vi "measure RTD (host).vi"() -> ()   [LabVIEW 2012]
uses:
  <vilib>/FPGAPlugInAG/PCIe-7852R/niLvFpga_Open_PCIe-7852R.vi
  <vilib>/rvi/interface/common/dynamic/niFpgaDynamicAddResources.vi
  <vilib>/Utility/error.llb/Error Cluster From Error Code.vi
  <vilib>/rvi/errors/niLvFpgaAdjustHostInterfaceError.vi
  <vilib>/rvi/interface/nirviOpenFPGA/nirviOpenFPGA.xnode
  FPGA Bitfiles/UHR-FleezersInst_FPGATarget_rtdmeasure(fpga)_zG2qwe5Jbpg.lvbitx
  rtd measure (fpga).vi
  <vilib>/rvi/interface/nirviReadWriteControl/nirviReadWriteControl.xnode
  NiFpgaLv.dll
  <vilib>/rvi/interface/Simulation/niFpgaSimulationCallBeginRW.vi
panel:
  out "Temp Var":dbl[][](graph) caption="Temperature Variation (F) (initial temp subtracted)"
  out "Absolute Temperature (F)":dbl[][](graph)
  out "Temp (F)":dbl[](array[numeric])
  out "Temp (C)":dbl[](array[numeric])
  out "Resistance":fxp<+/-,24,10>[](array[numeric])
  out "Path Out":path
  out "Index In":dbl=1.0
  in  "Save the data":bool
  in  "stop":bool
  in  "milliseconds to wait":u32=100
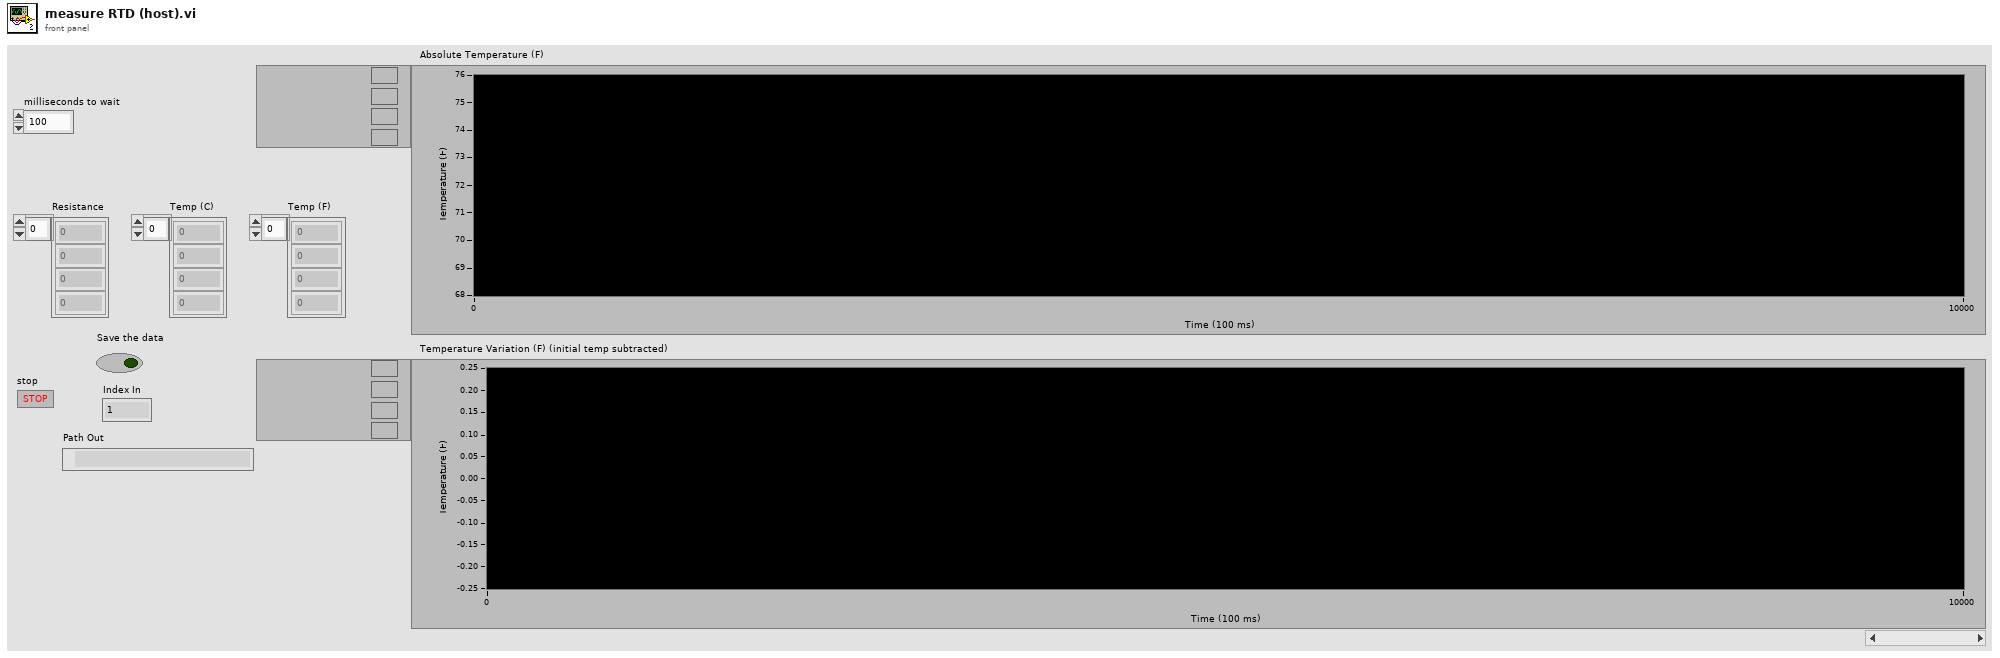
[diagram p1: front panel]
types:
  T1 = enum16{"big-endian, network order", "native, host order", "little-endian"}
  T2 = enum16{"open", "replace", "create", "open or create", "replace or create", "replace or create with confirmation"}
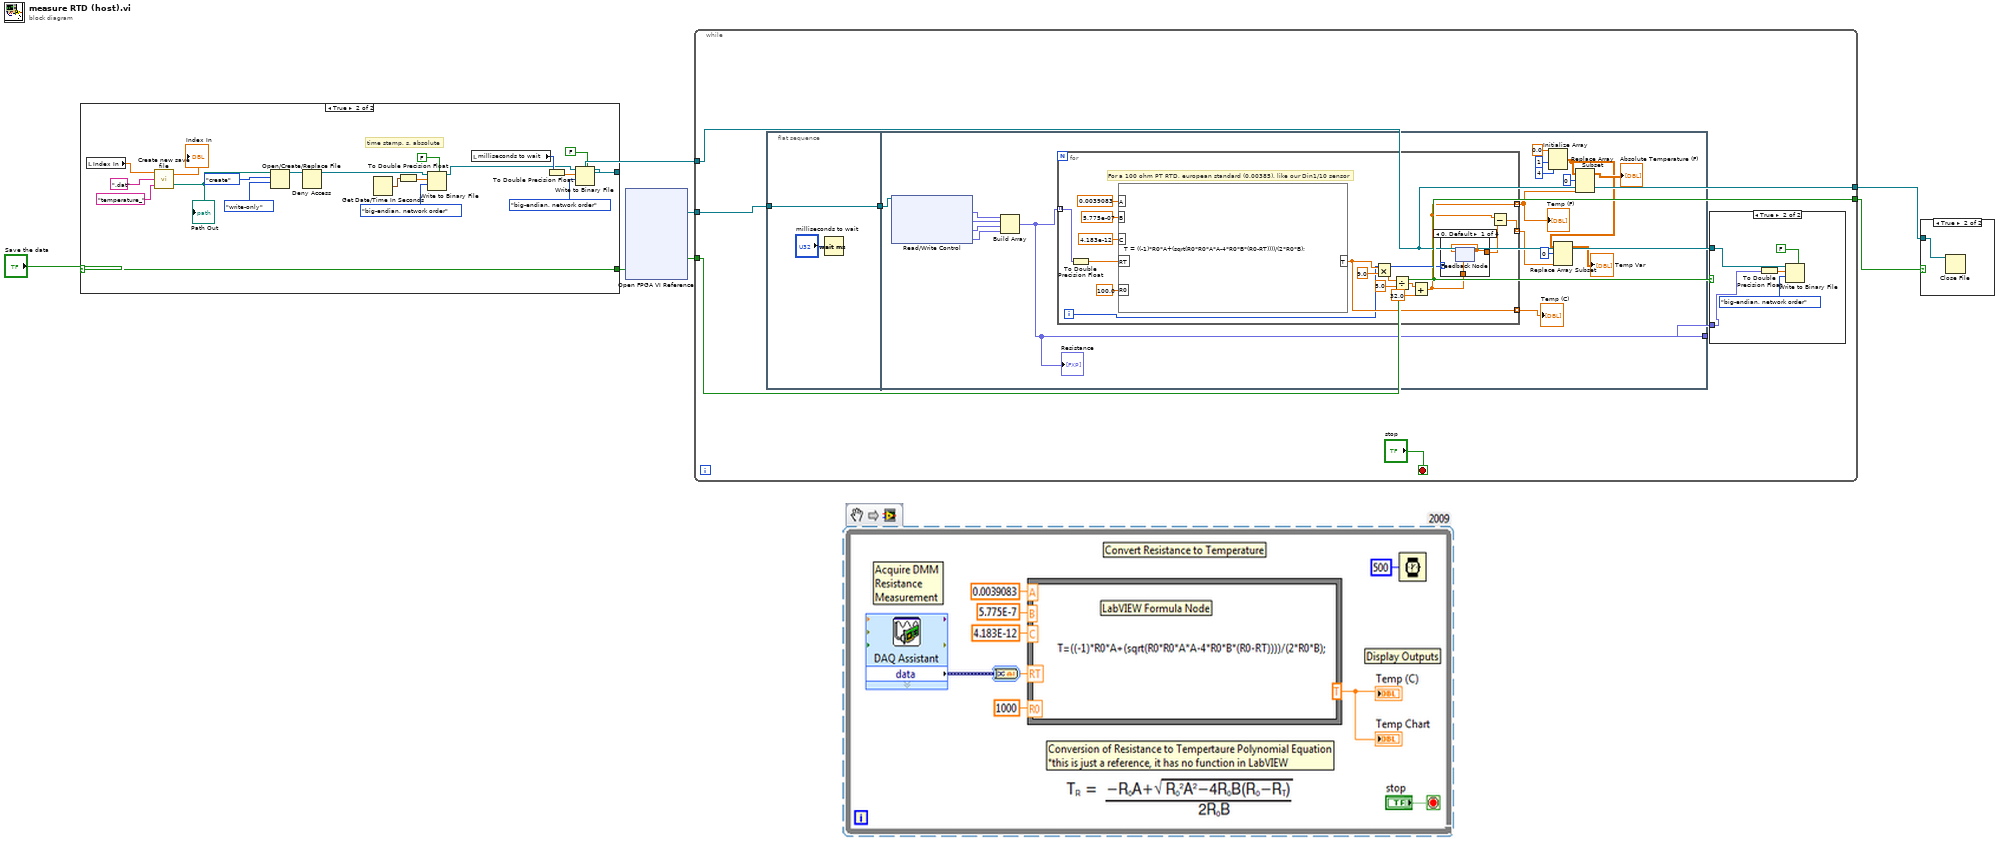
[diagram p0: block diagram]
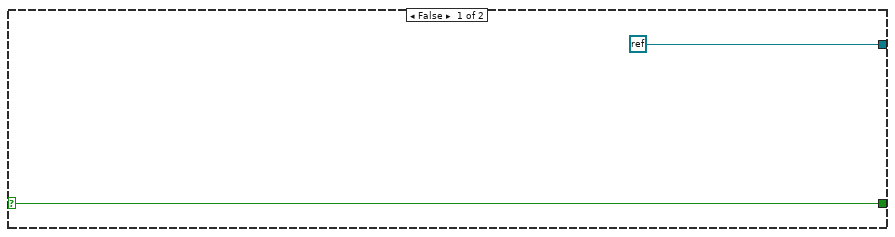
[diagram p3: hidden frame]
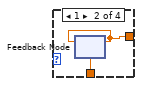
[diagram p5: hidden frame]
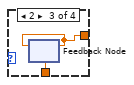
[diagram p6: hidden frame]
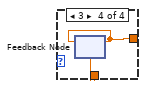
[diagram p7: hidden frame]
diagram:
  n1 = case shown="True" "Save the data" {
    selector: "Save the data" -> [w8 w20]
    tunnel: [w8 w20] -> w4
    tunnel: [refnum<k0> refnum w17] -> w3
    frame False {
    }
    frame True {
      # "time stamp, s, absolute"
      n2 = local read "Index In"() -> (w27:dbl)
      n3 = call "Create new save file.vi"("Insert"="temperature_", "Ext"=".dat", "Index In"=w27) -> ("Path Out"=w24:path, "Index Out"=→"Index In":dbl)
      "Path Out" <- w24
      n4 = Open/Create/Replace File(file path (use dialog)=w24, operation (0:open)=T2."create", access (0:read/write)=enum16{"read/write", "read-only", "write-only"}."write-only") -> (refnum out=w21:refnum<file>)  [unwired: 1 in, 4 out]
      n5 = Deny Access(7:w21) -> (3:w11:refnum<file>)  [unwired: 1 in, 2 out]
      n6 = Get Date/Time In Seconds() -> (seconds since 1Jan1904=w9:timestamp)
      n7 = To Double Precision Float(number=w9) -> (double precision float=w12:dbl)
      n8 = Write to Binary File(file (use dialog)=w11, data=w12, 5:FALSE ("prepend array or string size? (T)"), 9:T1."big-endian, network order" ("byte order (0:big-endian, network order)")) -> (refnum out=w10:refnum<file>)  [unwired: 1 in, 3 out]
      n9 = local read "milliseconds to wait"() -> (w16:u32)
      n10 = To Double Precision Float(number=w16) -> (double precision float=w15:dbl)
      n11 = Write to Binary File(file (use dialog)=w10, data=w15, 5:FALSE ("prepend array or string size? (T)"), 9:T1."big-endian, network order" ("byte order (0:big-endian, network order)")) -> (refnum out=w17:refnum<file>)  [unwired: 1 in, 3 out]
    }
  }
  n12 = xnode "Open FPGA VI Reference"() -> ("FPGA VI Reference Out"=w6:refnum<k20>)  [unwired: 2 in, 1 out]
  n13 = while {
    tunnel: w6 -> [w33]
    tunnel: w4 -> [w31]
    tunnel: w3 -> [w30]
    tunnel: [w31] -> w2
    tunnel: [w30] -> w1
    stop <- "stop" stop-if-true
    n14 = flat-sequence {
      tunnel: [w40] -> w34
      tunnel: w33 -> [w40]
      tunnel: w34 -> [w58]
      tunnel: [w53] -> w29
      frame #0 {
        n15 = Wait (ms)(milliseconds to wait="milliseconds to wait") -> ()  [unwired: 1 out]
      }
      frame #1 {
        n16 = xnode "Read/Write Control"("FPGA VI Reference In"=w58) -> ("Chassis2/Mod3/RTD0"=w57:fxp<+/-,24,10>, "Chassis2/Mod3/RTD1"=w56:fxp<+/-,24,10>, "Chassis2/Mod3/RTD2"=w55:fxp<+/-,24,10>, "Chassis2/Mod3/RTD3"=w54:fxp<+/-,24,10>)  [unwired: 1 in, 2 out]
        n17 = Build Array(w57, w56, w55, w54) -> (w53:fxp<+/-,24,10>[])
        "Resistance" <- w53
        n18 = for {
          tunnel: w53 -> [w64] mode=indexing
          tunnel: [w63] -> w48 mode=indexing
          tunnel: [w61] -> w46 mode=indexing
          tunnel: [w59] -> w43 mode=indexing
          i -> [w62]
          # "For a 100 ohm PT RTD, european standard (0.00385), like our Din1/10 sensor"
          n19 = To Double Precision Float(number=w64) -> (double precision float=w71:dbl)
          n20 = formula code="T = ((-1)*R0*A+(sqrt(R0*R0*A*A-4*R0*B*(R0-RT))))/(2*R0*B);"("A"=0.0039083 ("input variable"), "B"=5.775e-07 ("input variable"), "C"=4.183e-12 ("input variable"), "RT"=w71, "R0"=100.0 ("input variable")) -> ("T"=w63:dbl)
          n21 = Multiply(x=w63, y=9.0) -> (x*y=w68:dbl)
          n22 = Divide(x=w68, y=5.0) -> (x/y=w66:dbl)
          n23 = Add(x=w66, y=32.0) -> (x+y=w61:dbl)
          n24 = case shown="0, Default" w62 {
            tunnel: w61 -> [w76 w78 w80 w82]
            tunnel: [w75 w77 w79 w81] -> w60
            frame 0, Default {
              n25 = feedback #1(w76) -> (w75:dbl)
              n26 = feedback-in #1(w75) -> ()
            }
            frame 1 {
              n27 = feedback #2(w78) -> (w77:dbl)
              n28 = feedback-in #2(w77) -> ()
            }
            frame 2 {
              n29 = feedback #3(w80) -> (w79:dbl)
              n30 = feedback-in #3(w79) -> ()
            }
            frame 3 {
              n31 = feedback #4(w82) -> (w81:dbl)
              n32 = feedback-in #4(w81) -> ()
            }
          }
          n33 = Subtract(x=w61, y=w60) -> (x-y=w59:dbl)
        }
        "Temp (C)" <- w48
        "Temp (F)" <- w46
        n34 = Initialize Array(0.0 ("element"), 1 ("dimension size"), 4 ("dimension size")) -> (w44:dbl[][])
        n35 = Replace Array Subset(array=w44, new element=w43, index (row)=0) -> (→"Temp Var":dbl[][])  [unwired: 1 in]
        n36 = Replace Array Subset(array=w44, new element=w46, index (row)=0) -> (→"Absolute Temperature (F)":dbl[][])  [unwired: 1 in]
      }
    }
    n37 = case shown="True" w31 {
      tunnel: w30 -> [_ w39]
      tunnel: w29 -> [_ w35]
      frame False {
      }
      frame True {
        n38 = To Double Precision Float(number=w35) -> (double precision float=w36:dbl[])
        n39 = Write to Binary File(file (use dialog)=w39, data=w36, 5:FALSE ("prepend array or string size? (T)"), 9:T1."big-endian, network order" ("byte order (0:big-endian, network order)")) -> ()  [unwired: 1 in, 4 out]
      }
    }
  }
  n40 = case shown="True" w2 {
    tunnel: w1 -> [_ w83]
    frame False {
    }
    frame True {
      n41 = Close File(refnum=w83) -> ()  [unwired: 1 in, 2 out]
    }
  }
